vi "Message Timer.vi"(3 "Error In":errorcluster, 4 "Reset?":bool) -> (0 "Error Out":errorcluster, 1 "Timer Count":u32)   [LabVIEW 2018]
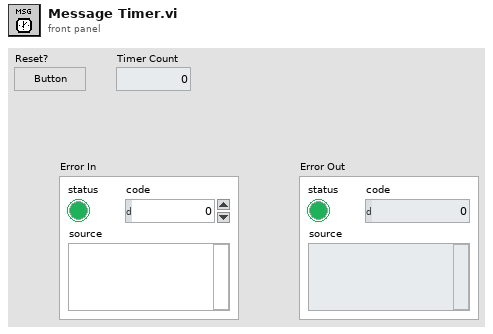
[diagram p1: front panel]
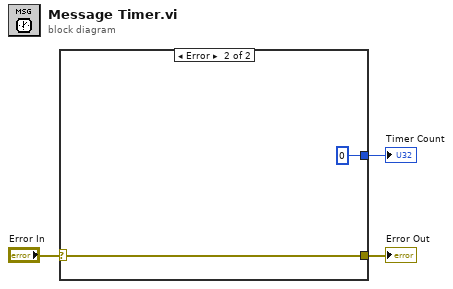
[diagram p0: block diagram]
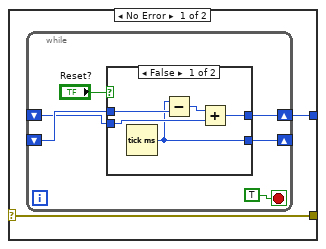
[diagram p2: hidden frame]
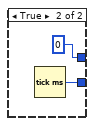
[diagram p3: hidden frame]
diagram:
  n1 = case shown="Error" "Error In" {
    selector: "Error In" -> [w4 w19]
    tunnel: [w5 u32 0 ("millisecond timer value")] -> w2
    tunnel: [w4 w19] -> w1
    frame No Error {
      n2 = while {
        shift-right: [w9] -> w5
        shift-left: _ -> [w6]
        shift-right: [w8] -> _
        shift-left: _ -> [w7]
        stop <- TRUE stop-if-true
        n3 = case shown="False" "Reset?" {
          tunnel: [w13 u32 0 ("millisecond timer value")] -> w9
          tunnel: [w12 w18] -> w8
          tunnel: w7 -> [w16 _]
          tunnel: w6 -> [w14 _]
          frame False {
            n4 = Tick Count (ms)() -> (millisecond timer value=w12:u32)
            n5 = Subtract(x=w12, y=w16) -> (x-y=w15:u32)
            n6 = Add(x=w15, y=w14) -> (x+y=w13:u32)
          }
          frame True {
            n7 = Tick Count (ms)() -> (millisecond timer value=w18:u32)
          }
        }
      }
    }
    frame Error {
    }
  }
  "Error Out" <- w1
  "Timer Count" <- w2
